vi "Befehl senden.vi"(11 "connection ID":refnum<k5>) -> (0 "error out":errorcluster, 2 "Verknüpfter String":string, 3 "connection ID":refnum<k5>)   [LabVIEW 2020, in "FT-IR.lvlib" / "AK-Interface.lvlib"]
uses:
  AK-Interface.lvlib
  Kommandos verwalten Aktionen.ctl
  TCP Timeout Aktionen - FTIR.ctl
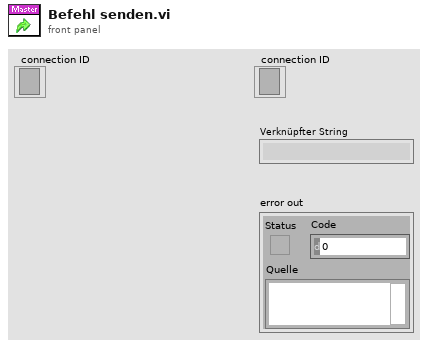
[diagram p1: front panel]
types:
  T1 = typedef "FT-IR.lvlib/AK-Interface.lvlib/TCP Timeout Aktionen - FTIR.ctl" = enum16{"lesen", "setzen"}
  T2 = typedef "FT-IR.lvlib/AK-Interface.lvlib/Kommandos verwalten Aktionen.ctl" = enum16{"lesen", "setzen Ende", "setzen Pos1", "senden", "initalisieren", "prüfen", "Kommandos"}
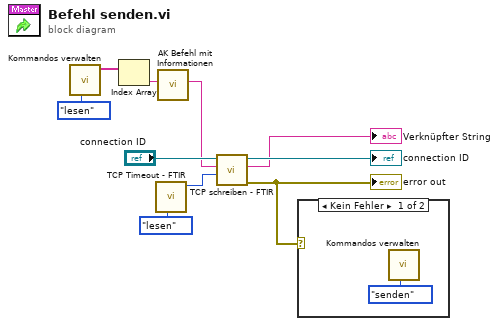
[diagram p0: block diagram]
diagram:
  n1 = call "Kommandos verwalten.vi"("Aktionen"=Kommandos_verwalten_Aktionen."lesen") -> ("Kommandos"=w3:string[])  [unwired: 8 in, 2 out]
  n2 = Index Array(array=w3) -> (element=w5:string)  [unwired: 1 in]
  n3 = call "TCP Timeout - FTIR.vi"("Aktionen Timeout"=TCP_Timeout_Aktionen_-_FTIR."lesen") -> ("Timeout schreiben"=w2:i32)  [unwired: 9 in, 1 out]
  n4 = call "AK Befehl mit Informationen.vi"("AK Befehl"=w5) -> ("String für schreiben"=w4:string)  [unwired: 10 in]
  n5 = call "TCP schreiben - FTIR.vi"("Timeout schreiben"=w2, "String"=w4, "connection ID"="connection ID") -> ("error out"=w7:errorcluster, "Verknüpfter String"=→"Verknüpfter String":string, "connection ID"=→"connection ID":refnum<k5>)  [unwired: 6 in]
  "error out" <- w7
  n6 = case shown="Kein Fehler" w7 {
    frame No Error {
      n7 = call "Kommandos verwalten.vi"("Aktionen"=Kommandos_verwalten_Aktionen."senden") -> ()  [unwired: 8 in, 3 out]
    }
    frame Error {
    }
  }
